vi "Query.vi"(8 "error in":errorcluster, 10 "Query":string, 11 "DB-MySQL in":refnum<class "DB-MySQL.lvclass">=refnum) -> (0 "error out":errorcluster, 1 "Packet Metadata":variant, 2 "Return Data":string[][](array[string]), 3 "DB-MySQL out":refnum<class "DB-MySQL.lvclass">, 4 "Field Names":string[](array[string]))   [LabVIEW 2014, in "hse-db.lvlib" / "DB-MySQL.lvclass"]
uses:
  DB-MySQL.lvclass
  DB-MySQL.lvclass/DB-MySQL.ctl
  DB-Engines/MySQLTcp/MySQL (TCP).lvlib
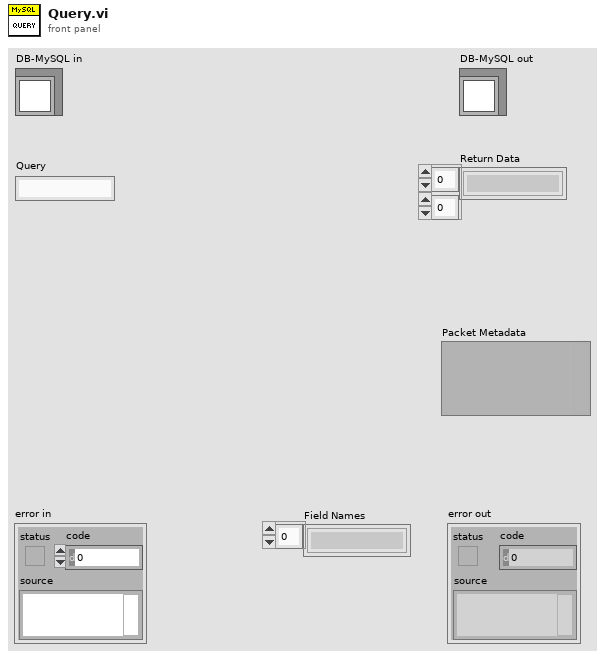
[diagram p1: front panel]
types:
  T1 = typedef "hse-db.lvlib/MySQL (TCP).lvlib/OK Packet Metadata.ctl" = cluster{"Affected Rows":u64, "Insert ID":u64, "Server Status":u16, "Warning Count":u16, "Message":string}
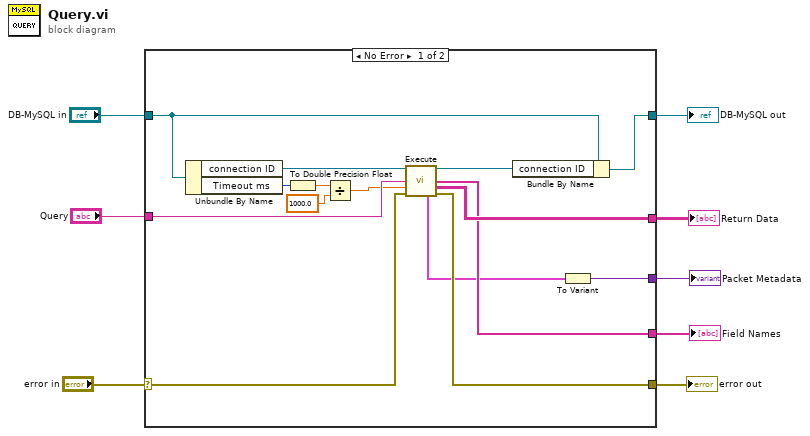
[diagram p0: block diagram]
diagram:
  n1 = case shown="No Error" "error in" {
    selector: "error in" -> [w21 w24]
    tunnel: "Query" -> [w18 _]
    tunnel: [w22 w25] -> w5
    tunnel: "DB-MySQL in" -> [w23 w25]
    tunnel: [w20 w24] -> w4
    tunnel: [w16 _] -> w2
    tunnel: [w15 _] -> w3
    tunnel: [w9 _] -> w1
    frame No Error {
      n2 = Unbundle By Name(w23) -> ("connection ID"=w19:refnum<k5>, "Timeout ms"=w14:i32)
      n3 = To Double Precision Float(number=w14) -> (double precision float=w13:dbl)
      n4 = Divide(x=w13, y=1000.0) -> (x/y=w11:dbl)
      n5 = call "Execute.vi"("connection ID in"=w19, "Query"=w18, "Timeout (60s)"=w11, "error in (no error)"=w21) -> ("connection ID out"=w17:refnum<k5>, "Field Names"=w15:string[], "Recordset data out"=w16:string[][], "Packet Metadata"=w10:T1, "error out"=w20:errorcluster)  [unwired: 6 in, 1 out]
      n6 = Bundle By Name(cluster=w23, "connection ID"=w17) -> (w22:refnum<class "DB-MySQL.lvclass">)
      n7 = To Variant(anything=w10) -> (Variant=w9:variant)
    }
    frame Error {
    }
  }
  "error out" <- w4
  "DB-MySQL out" <- w5
  "Field Names" <- w3
  "Return Data" <- w2
  "Packet Metadata" <- w1
